vi "Default Settings.vi"(8 "error in (no error)":errorcluster, 11 "CAD Dispense in":refnum<class "Sensor Dispense.lvclass">) -> (0 "error out":errorcluster, 3 "CAD Dispense out":refnum<class "Sensor Dispense.lvclass">)   [LabVIEW 2016, in "Sensor Dispense.lvclass"]
uses:
  Sensor Dispense.lvclass
  C:/Users/HEP Gantry/Documents/GitHub/UCSB-Gantry/V5/Classes/Routine/Dispense/Dispense.lvclass
  Sensor Dispense.lvclass/Sensor Dispense.ctl
  Dispense.lvclass/Dispense.ctl
  Write Tip Height.vi
panel:
  # "This Routine does not Accept Settings"
  # "This Routine Does not Accept Settings"
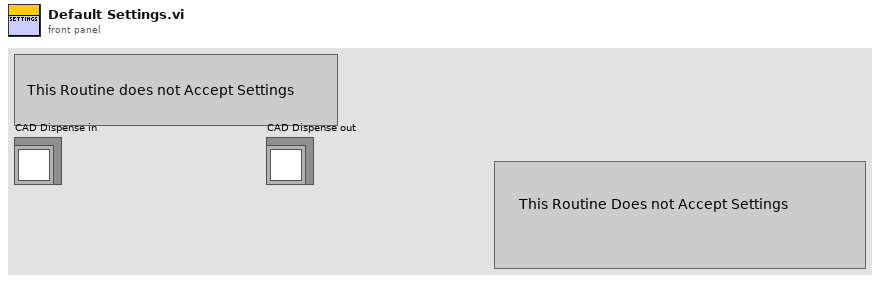
[diagram p1: front panel]
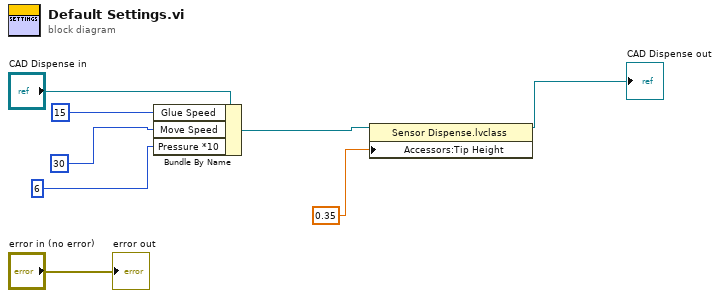
[diagram p0: block diagram]
diagram:
  n1 = Bundle By Name(cluster="CAD Dispense in", "Glue Speed"=15, "Move Speed"=30, "Pressure *10"=6) -> (w3:refnum<class "Sensor Dispense.lvclass">)
  n2 = property class="Sensor Dispense.lvclass"(reference=w3, "Accessors:Tip Height"=0.35) -> (reference out=→"CAD Dispense out":refnum<class "Sensor Dispense.lvclass">)  [unwired: 1 in, 1 out]
  "error out" <- "error in (no error)"
